vi "Recipe.vi"() -> ()   [LabVIEW 2020, in "SMCD14_lib.lvlib"]
uses:
  SMCD14_lib.lvlib
  Macro Cluster.ctl
  typedefAxisConfiguration.ctl
  ConnectionData.vi
  AxisWriteValues.vi
  AxisWriteValues_Write.vi
panel:
  out "AxisBaseAddr":u16[](array[numeric])
  in  "Macro Table":T1[](array[typedef]) {"M5_select_action" items=["Stop", "Safe Position", "Working Position", "Run scaning", "Transfer posituin"]; "SelectedTargetCtrl" items=["none", "Target 1", "Target 2", "Target 3", "Target 4", "Target 5", "Target 6", "Laser test"]; "M3_Type" items=["Type1", "Type2", "Type3", "Type4", "Type5"]; "M3_1_Time" format="%<%H:%M:%S>t"; "MoveModeControl" items=["Absolute"=1, "Relative"=2, "Velocity"=3, "Homing"=4, "none"=0]; "M2_Target_Vel" format="%<%H:%M:%S>t"; "M2_Axis" items=["Axis no1", "Axis no2", "Axis no3", "Axis no4", "Axis no5", "Axis no6"]; "M1_action_axis 6" items=["NONE", "Start", "Stop", "Clear", "Motor ON", "motor OFF"]; "M1_action_axis 5" items=["NONE", "Start", "Stop", "Clear", "Motor ON", "motor OFF"]; "M1_action_axis 4" items=["NONE", "Start", "Stop", "Clear", "Motor ON", "motor OFF"]; "M1_action_axis 3" items=["------", "Manual", "Time SP", "Thickness SP"]; "M1_action_axis 2" items=["NONE", "Start", "Stop", "Clear", "Motor ON", "motor OFF"]; "M1_action_axis 1" items=["NONE", "Start", "Stop", "Clear", "Motor ON", "motor OFF"]; "Macro Type" items=["Action", "Parameters", "Wait"]}
  out "AxisNames":string[](array[string])
  out "Recipe example":refnum<vi>
  in  "AxisControlSubPanelRefArray":refnum<vi>[](array[refnum])
  in  "AxesCount":i32=6
  out "AllowCalib":bool
  out "Act. macro:":string
  out "Recipe Finish:":bool
  out "Recipe in Progress:":bool
  out "?":cluster{dbl, dbl}(slide)={-100.0, 0.0} scale=0.0..100.0 scale format="%.0f %"
  out "Act. Step:":i32=-1
  in  "Stop Recipe":bool
  in  "Start Recipe":bool
  in  "Next macro":bool
  in  "E. Recipe":bool=TRUE
  out "MacroStart Time":timestamp
  out "Act. Macro:":i32=-1
  out "SlavesID":u16[](array[numeric])
  out "size":i32=1
  out "New Macro":bool
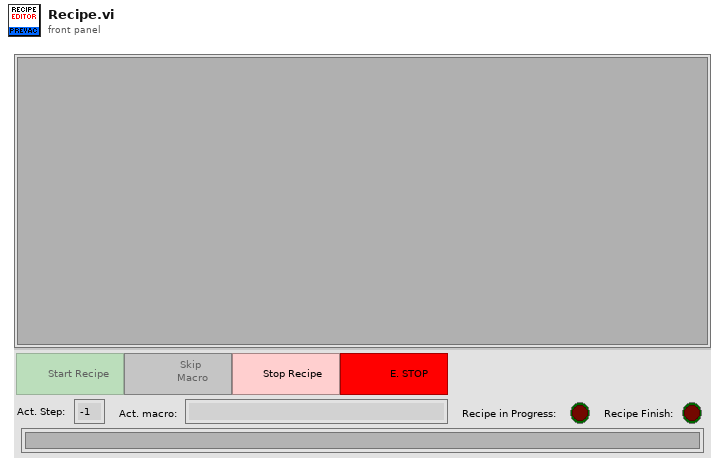
[diagram p1: front panel]
types:
  T1 = typedef "SMCD14_lib.lvlib/Macro Cluster.ctl" = cluster{"Macro Type":u16, "Macro Name":string, "Macro Description":string, "M1_action_axis 1":u16, "M1_action_axis 2":u16, "M1_action_axis 3":u16, "M1_action_axis 4":u16, "M1_action_axis 5":u16, "M1_action_axis 6":u16, "M2_Axis":u16, "M2_Target_Pos":sgl, "M2_Target_Vel":sgl, "MoveModeControl":u16, "M3_1_Time":u32, "M3_Type":u16, "M3_2_wait_for_axis 1":bool, "M3_2_wait_for_axis 2":bool, "M3_2_wait_for_axis 3":bool, "M3_2_wait_for_axis 4":bool, "M3_2_wait_for_axis 5":bool, "M3_2_wait_for_axis 6":bool, "M3_3_mesage":string, "M3_3_wait_for_calib":bool, "SelectedTargetCtrl":u16, "M5_select_action":u16}
  T2 = typedef "SMCD14_lib.lvlib/AxisWriteValues_typedef.ctl" = cluster{"AxisTarget":dbl, "AxisTargetVel":dbl, "AxisStartReq":bool, "AxisStopReq":bool, "AxisClearReq":bool, "AxisMovetype":bool, "AxisMotorON":bool, "MoveModeControl":u16, "AxisHomingVel":dbl, "AxisAccDecc":dbl}
  T3 = enum16{"Left Button", "Center Button", "Right Button", "Window Close"}
  T4 = enum8{"Enabled", "Disabled", "Disabled and Grayed Out"}
  T5 = typedef "SMCD14_lib.lvlib/ConnectionData_typedef.ctl" = cluster{"DeviceIDCtrl":u16, "ProtocolCtrl":enum16{"Modbus RTU", "Modbus TCP", ""}, "COMportCtrl":refnum<visa-resource-name>, "IPCtrl":string, "serial master instance":refnum<class "Modbus Master.lvclass">, "ConnectionStatusIndicator":bool}
  T6 = typedef "SMCD14_lib.lvlib/typedefAxisConfiguration.ctl" = cluster{"AxisName":string, "UnitsControl":u16, "AxisSlaveID":u16, "AxisBaseAddr":u16, "AxisMinSpeed":dbl, "AxisMaxSpeed":dbl}
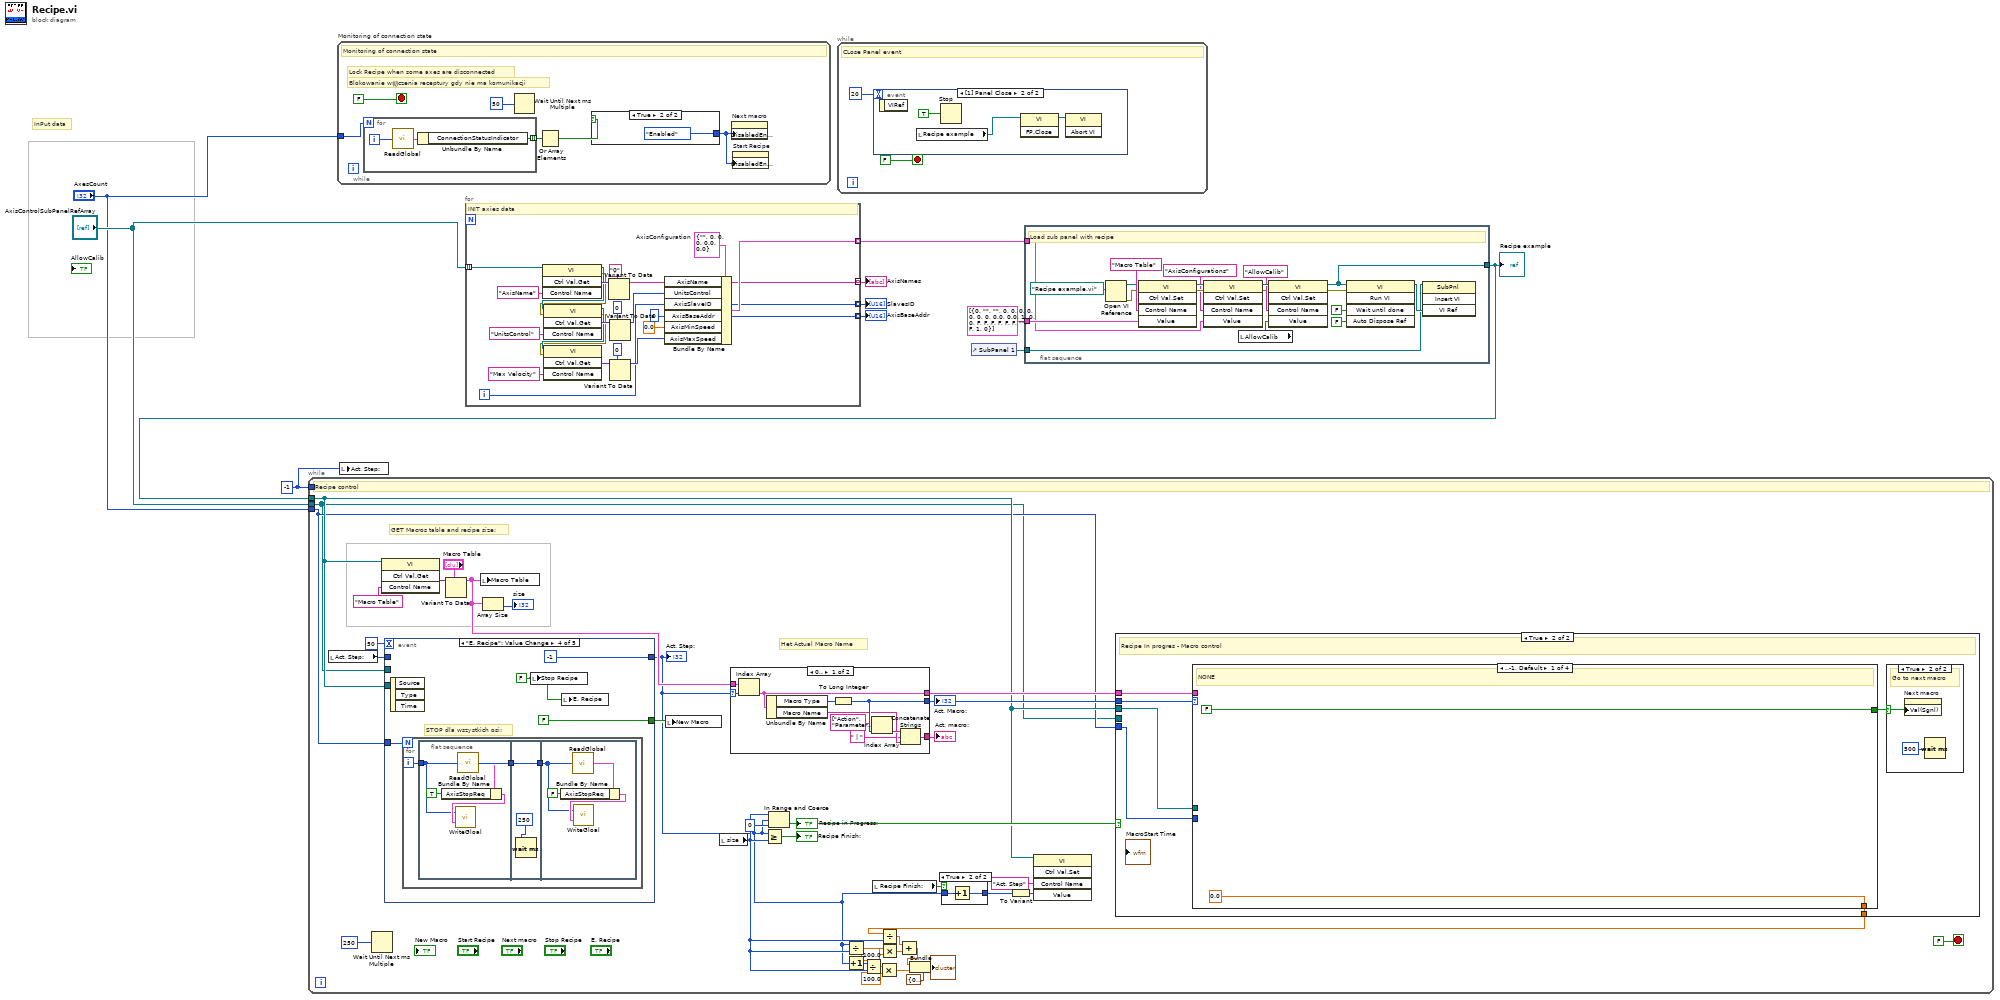
[diagram p0: block diagram]
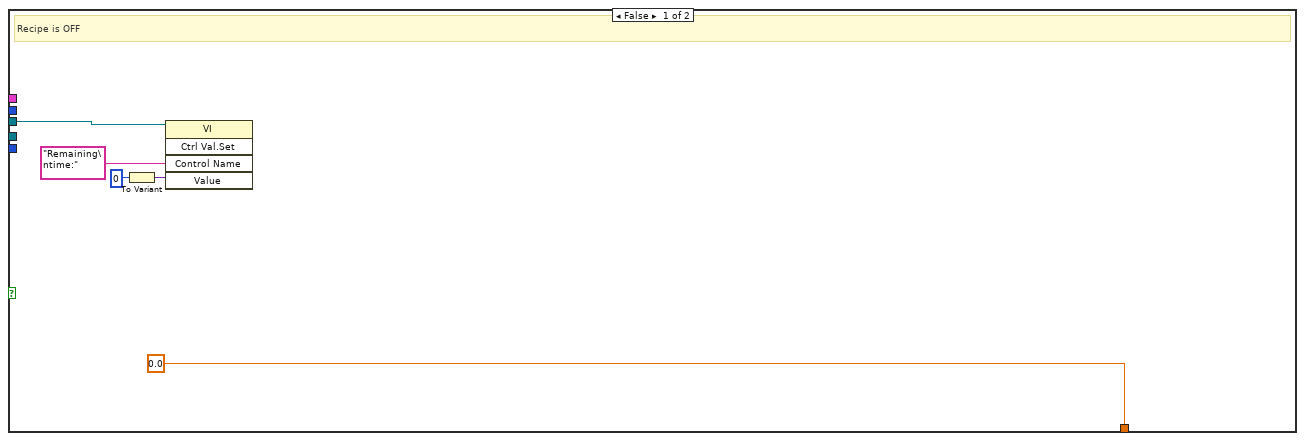
[diagram p3: hidden frame]
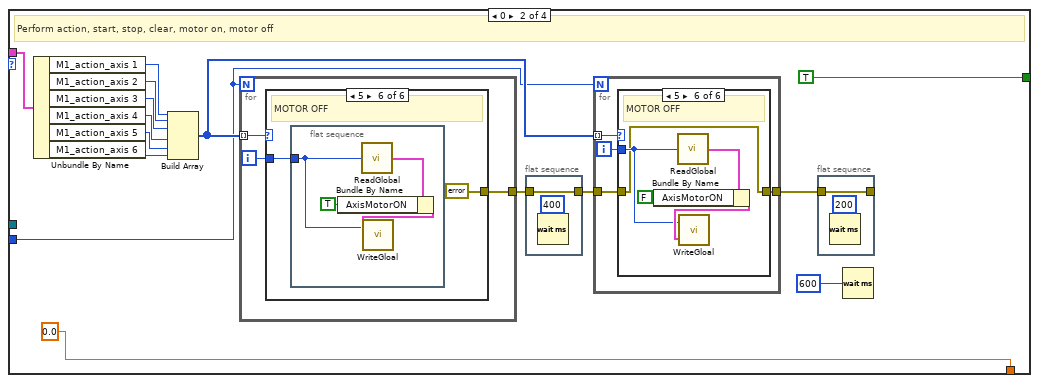
[diagram p5: hidden frame]
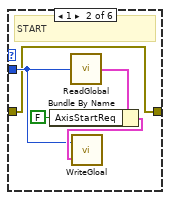
[diagram p7: hidden frame]
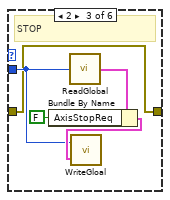
[diagram p8: hidden frame]
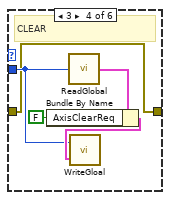
[diagram p9: hidden frame]
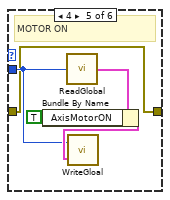
[diagram p10: hidden frame]
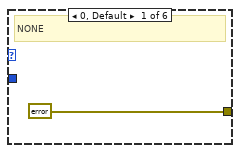
[diagram p11: hidden frame]
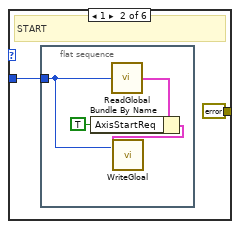
[diagram p12: hidden frame]
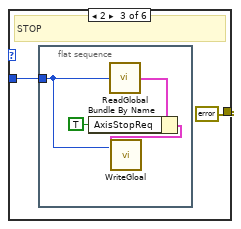
[diagram p13: hidden frame]
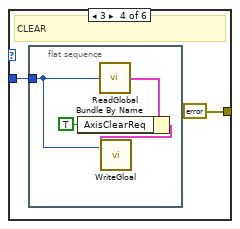
[diagram p14: hidden frame]
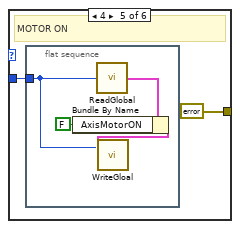
[diagram p15: hidden frame]
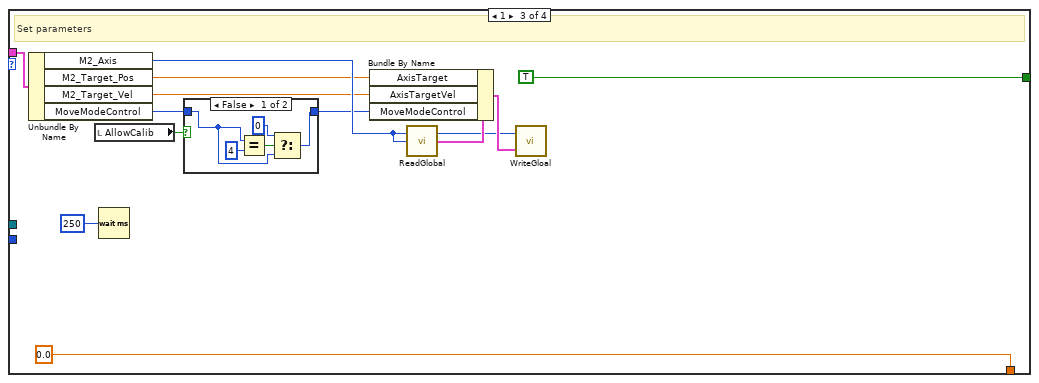
[diagram p16: hidden frame]
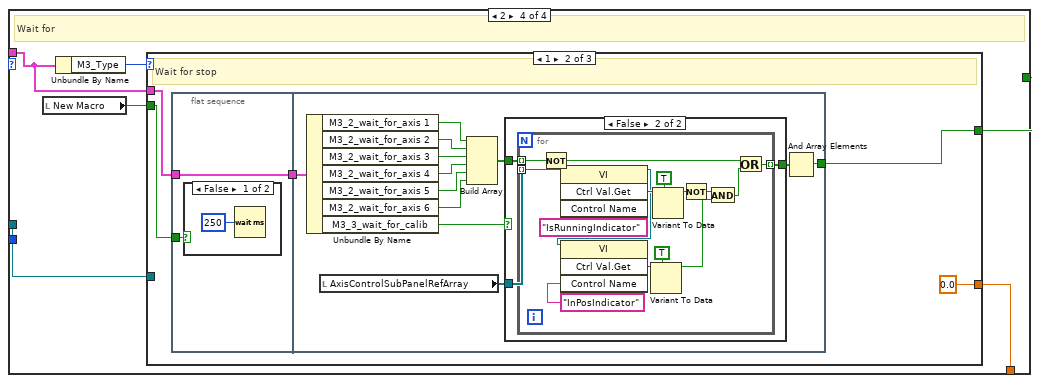
[diagram p18: hidden frame]
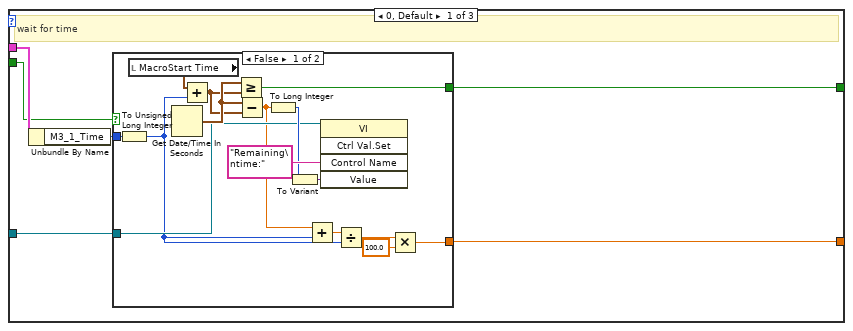
[diagram p19: hidden frame]
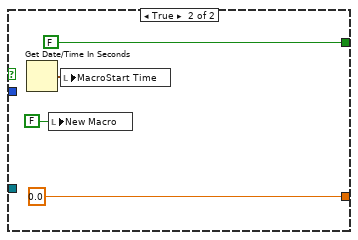
[diagram p20: hidden frame]
diagram:
  w7 = -1
  # "InPut data"
  n1 = while {
    tunnel: w4 -> [w15]
    tunnel: w7 -> [_]
    tunnel: "AxisControlSubPanelRefArray" -> [w11]
    tunnel: "AxesCount" -> [w12]
    stop <- FALSE stop-if-true
    # "Het Actual Macro Name"
    # "GET Macros table and recipe size:"
    # "Recipe control"
    n2 = local read "Act. Step:"() -> (w46:i32)
    n3 = Wait Until Next ms Multiple(millisecond multiple=u32 250) -> ()  [unwired: 1 out]
    n4 = invoke class="VI" method="Ctrl Val.Get"(reference=w15, "Control Name"="Macro Table") -> ("Get Control Value Variant"=w40:variant)  [unwired: 2 in, 3 out]
    n5 = event shown="[3] \"E. Recipe\": Value Change" {
      selector: _ -> [_ _ _ _ _]
      dyn-events: _ -> [_ _ _ _ _]
      timeout: 50 -> [_ _ _ _ _]
      tunnel: w46 -> [w281 _ _ _ w314]
      tunnel: [w280 0 ("millisecond multiple") -1 ("millisecond multiple") -1 ("millisecond multiple") w312] -> w13
      tunnel: [w287 TRUE ("Play Button") FALSE ("Play Button") FALSE ("Play Button") TRUE ("New Macro")] -> w43
      tunnel: w11 -> [_ _ _ _ _]
      tunnel: w15 -> [w284 _ _ _ _]
      tunnel: w12 -> [_ _ _ w294 _]
      event Timeout {
        n6 = event-data() -> ()  [unwired: 1 in, 3 out]
        n7 = local read "Recipe in Progress:"() -> (w279:bool)
        n8 = invoke class="VI" method="Ctrl Val.Get"(reference=w284, "Control Name"="edit?") -> ("Get Control Value Variant"=w286:variant)  [unwired: 2 in, 3 out]
        n9 = Variant To Data(type=FALSE ("Play Button"), Variant=w286) -> (data=w277:bool)  [unwired: 1 in, 1 out]
        n10 = Not(x=w279) -> (.not. x?=w278:bool)
        n11 = local read "New Macro"() -> (w287:bool)
        n12 = And(x=w278, y=w277) -> (x .and. y?=w276:bool)
        n13 = Select(t=-1, s=w276, f=w281) -> (s? t:f=w280:i32)
      }
      event "Start Recipe": Value Change {
        n14 = event-data() -> ()  [unwired: 1 in, 3 out]
        n15 = local write "Start Recipe"(FALSE ("Play Button")) -> ()
      }
      event "Stop Recipe": Value Change {
        n16 = event-data() -> ()  [unwired: 1 in, 3 out]
        n17 = local write "Stop Recipe"(FALSE ("Play Button")) -> ()
      }
      event "E. Recipe": Value Change {
        w295 = FALSE ("Play Button")
        # "STOP dla wszystkich osi:"
        n18 = event-data() -> ()  [unwired: 1 in, 3 out]
        n19 = for {
          N: w294 -> [_]
          i -> [w298]
          n20 = flat-sequence {
            tunnel: w298 -> [w302]
            tunnel: [w302] -> w300
            tunnel: w300 -> [w305]
            tunnel: [w305] -> w299
            tunnel: w299 -> [w307]
            frame #0 {
              n21 = call-poly "ReadGlobal.vi"("AxisNo"=w302) -> ("AxisWriteValuesOUT"=w301:T2)
              n22 = Bundle By Name(cluster=w301, "AxisStopReq"=TRUE ("AxisWriteValues.AxisMotorON")) -> (w303:T2)
              n23 = call-poly "WriteGloal.vi"("AxisWriteValuesIN"=w303, "AxisNo"=w302) -> ()  [unwired: 1 in]
            }
            frame #1 {
              n24 = Wait (ms)(milliseconds to wait=u32 250) -> ()  [unwired: 1 out]
            }
            frame #2 {
              n25 = call-poly "ReadGlobal.vi"("AxisNo"=w307) -> ("AxisWriteValuesOUT"=w309:T2)
              n26 = Bundle By Name(cluster=w309, "AxisStopReq"=FALSE ("AxisWriteValues.AxisMotorON")) -> (w308:T2)
              n27 = call-poly "WriteGloal.vi"("AxisWriteValuesIN"=w308, "AxisNo"=w307) -> ()  [unwired: 1 in]
            }
          }
        }
        n28 = local write "Stop Recipe"(w295) -> ()
        n29 = local write "E. Recipe"(w295) -> ()
      }
      event "Next macro": Value Change {
        n30 = event-data() -> ()  [unwired: 1 in, 1 out]
        n31 = Greater Or Equal To 0?(x=w314) -> (x >= 0?=w318:bool)
        n32 = local read "size"() -> (w313:i32)
        n33 = case shown="True" w318 {
          tunnel: [w320 w322] -> w316
          tunnel: w314 -> [w320 w321]
          frame False {
          }
          frame True {
            n34 = Increment(x=w321) -> (x+1=w322:i32)
          }
        }
        n35 = Increment(x=w313) -> (x+1=w317:i32)
        n36 = In Range and Coerce(upper limit=w317, x=w316, lower limit=0 ("millisecond multiple")) -> (coerced(x)=w312:i32)  [unwired: 1 out]
        n37 = local write "Next macro"(FALSE ("Play Button")) -> ()
      }
    }
    "Act. Step:" <- w13
    n38 = Variant To Data(type="Macro Table", Variant=w40) -> (data=w26:T1[])  [unwired: 1 in, 1 out]
    n39 = local write "Macro Table"(w26) -> ()
    n40 = Array Size(array=w26) -> (size(s)=→"size":i32)
    n41 = local write "New Macro"(w43) -> ()
    n42 = local read "size"() -> (w14:i32)
    n43 = case shown="0.." w13 {
      selector: w13 -> [w272 _]
      tunnel: [w269 T1 {"Macro Type"=0, "Macro Name"="", "Macro Description"="", "M1_action_axis 1"=0, "M1_action_axis 2"=0, "M1_action_axis 3"=0, "M1_action_axis 4"=0, "M1_action_axis 5"=0, "M1_action_axis 6"=0, "M2_Axis"=0, "M2_Target_Pos"=0.0, "M2_Target_Vel"=0.0, "MoveModeControl"=0, "M3_1_Time"=0, "M3_Type"=0, "M3_2_wait_for_axis 1"=FALSE, "M3_2_wait_for_axis 2"=FALSE, "M3_2_wait_for_axis 3"=FALSE, "M3_2_wait_for_axis 4"=FALSE, "M3_2_wait_for_axis 5"=FALSE, "M3_2_wait_for_axis 6"=FALSE, "M3_3_mesage"="", "M3_3_wait_for_calib"=FALSE, "SelectedTargetCtrl"=1, "M5_select_action"=0} ("Macro Cluster")] -> w28
      tunnel: [w268 -1 ("millisecond multiple")] -> w25
      tunnel: w26 -> [w271 _]
      tunnel: [w263 "" ("Macro Name")] -> w24
      frame 0.. {
        n44 = Index Array(array=w271, index=w272) -> (element=w269:T1)
        n45 = Unbundle By Name(w269) -> ("Macro Type"=w270:u16, "Macro Name"=w265:string)
        n46 = To Long Integer(number=w270) -> (32bit integer=w268:i32)
        n47 = Index Array(array=string[] ["Action", "Parameters", "Wait"], index=w268) -> (element=w266:string)
        n48 = Concatenate Strings(w266, " | " ("string"), w265) -> (w263:string)
      }
      frame ..-1, Default {
      }
    }
    "Act. Macro:" <- w25
    "Act. macro:" <- w24
    n49 = Greater Or Equal?(x=w13, y=w14) -> (x >= y?=→"Recipe Finish:":bool)
    n50 = In Range and Coerce(upper limit=w14, x=w13, lower limit=0 ("millisecond multiple")) -> (In Range?=w29:bool)  [unwired: 1 out]
    "Recipe in Progress:" <- w29
    n51 = Divide(x=w13, y=w14) -> (x/y=w39:dbl)
    n52 = Increment(x=w13) -> (x+1=w33:i32)
    n53 = Divide(x=w33, y=w14) -> (x/y=w34:dbl)
    n54 = local read "Recipe Finish:"() -> (w17:bool)
    n55 = Multiply(x=w34, y=100.0) -> (x*y=w31:dbl)
    n56 = Multiply(x=w39, y=100.0) -> (x*y=w23:dbl)
    n57 = case shown="True" w17 {
      tunnel: w13 -> [w48 w50]
      tunnel: [w48 w49] -> w16
      frame False {
      }
      frame True {
        n58 = Increment(x=w50) -> (x+1=w49:i32)
      }
    }
    n59 = To Variant(anything=w16) -> (Variant=w19:variant)
    n60 = invoke class="VI" method="Ctrl Val.Set"(reference=w15, "Control Name"="Act. Step", "Value"=w19) -> ()  [unwired: 2 in, 5 out]
    n61 = case shown="True" w29 {
      tunnel: w28 -> [_ w59]
      tunnel: w25 -> [_ w61]
      tunnel: w15 -> [w52 w58]
      tunnel: [0.0 ("y") w57] -> w21
      tunnel: w12 -> [_ w56]
      tunnel: w11 -> [_ _]
      frame False {
        # "Recipe is OFF"
        n62 = To Variant(anything=0) -> (Variant=w55:variant)
        n63 = invoke class="VI" method="Ctrl Val.Set"(reference=w52, "Control Name"="Remaining\ntime:", "Value"=w55) -> ()  [unwired: 2 in, 5 out]
      }
      frame True {
        # "Recipe In progres - Macro control"
        n64 = case shown="..-1, Default" w61 {
          tunnel: [FALSE ("true") TRUE TRUE w167] -> w60
          tunnel: w59 -> [_ w80 w160 w170]
          tunnel: w58 -> [_ _ _ w169]
          tunnel: [0.0 0.0 0.0 w168] -> w57
          tunnel: w56 -> [_ w69 _ _]
          frame ..-1, Default {
            # "NONE"
          }
          frame 0 {
            # "Perform action, start, stop, clear, motor on, motor off"
            n65 = Unbundle By Name(w80) -> ("M1_action_axis 1"=w79:u16, "M1_action_axis 2"=w78:u16, "M1_action_axis 3"=w77:u16, "M1_action_axis 4"=w76:u16, "M1_action_axis 5"=w75:u16, "M1_action_axis 6"=w74:u16)
            n66 = Build Array(w79, w78, w77, w76, w75, w74) -> (w71:u16[])
            n67 = for {
              N: w69 -> [_]
              tunnel: w71 -> [w117] mode=indexing
              tunnel: [w116] -> w68
              i -> [w115]
              n68 = case shown="5" w117 {
                tunnel: [errorcluster {"status"=FALSE, "code"=0, "source"=""} ("error out") errorcluster {"status"=FALSE, "code"=0, "source"=""} ("error out") errorcluster {"status"=FALSE, "code"=0, "source"=""} ("error out") errorcluster {"status"=FALSE, "code"=0, "source"=""} ("error out") errorcluster {"status"=FALSE, "code"=0, "source"=""} ("error out") errorcluster {"status"=FALSE, "code"=0, "source"=""} ("error out")] -> w116
                tunnel: w115 -> [_ w120 w126 w132 w138 w144]
                frame 0, Default {
                  # "NONE"
                }
                frame 1 {
                  # "START"
                  n69 = flat-sequence {
                    tunnel: w120 -> [w121]
                    frame #0 {
                      n70 = call-poly "ReadGlobal.vi"("AxisNo"=w121) -> ("AxisWriteValuesOUT"=w123:T2)
                      n71 = Bundle By Name(cluster=w123, "AxisStartReq"=TRUE ("AxisWriteValues.AxisMotorON")) -> (w122:T2)
                      n72 = call-poly "WriteGloal.vi"("AxisWriteValuesIN"=w122, "AxisNo"=w121) -> ()  [unwired: 1 in]
                    }
                  }
                }
                frame 2 {
                  # "STOP"
                  n73 = flat-sequence {
                    tunnel: w126 -> [w127]
                    frame #0 {
                      n74 = call-poly "ReadGlobal.vi"("AxisNo"=w127) -> ("AxisWriteValuesOUT"=w129:T2)
                      n75 = Bundle By Name(cluster=w129, "AxisStopReq"=TRUE ("AxisWriteValues.AxisMotorON")) -> (w128:T2)
                      n76 = call-poly "WriteGloal.vi"("AxisWriteValuesIN"=w128, "AxisNo"=w127) -> ()  [unwired: 1 in]
                    }
                  }
                }
                frame 3 {
                  # "CLEAR"
                  n77 = flat-sequence {
                    tunnel: w132 -> [w133]
                    frame #0 {
                      n78 = call-poly "ReadGlobal.vi"("AxisNo"=w133) -> ("AxisWriteValuesOUT"=w135:T2)
                      n79 = Bundle By Name(cluster=w135, "AxisClearReq"=TRUE ("AxisWriteValues.AxisMotorON")) -> (w134:T2)
                      n80 = call-poly "WriteGloal.vi"("AxisWriteValuesIN"=w134, "AxisNo"=w133) -> ()  [unwired: 1 in]
                    }
                  }
                }
                frame 4 {
                  # "MOTOR ON"
                  n81 = flat-sequence {
                    tunnel: w138 -> [w139]
                    frame #0 {
                      n82 = call-poly "ReadGlobal.vi"("AxisNo"=w139) -> ("AxisWriteValuesOUT"=w141:T2)
                      n83 = Bundle By Name(cluster=w141, "AxisMotorON"=FALSE ("AxisWriteValues.AxisMotorON")) -> (w140:T2)
                      n84 = call-poly "WriteGloal.vi"("AxisWriteValuesIN"=w140, "AxisNo"=w139) -> ()  [unwired: 1 in]
                    }
                  }
                }
                frame 5 {
                  # "MOTOR OFF"
                  n85 = flat-sequence {
                    tunnel: w144 -> [w145]
                    frame #0 {
                      n86 = call-poly "ReadGlobal.vi"("AxisNo"=w145) -> ("AxisWriteValuesOUT"=w147:T2)
                      n87 = Bundle By Name(cluster=w147, "AxisMotorON"=TRUE ("AxisWriteValues.AxisMotorON")) -> (w146:T2)
                      n88 = call-poly "WriteGloal.vi"("AxisWriteValuesIN"=w146, "AxisNo"=w145) -> ()  [unwired: 1 in]
                    }
                  }
                }
              }
            }
            n89 = flat-sequence {
              tunnel: w68 -> [w83]
              tunnel: [w83] -> w67
              frame #0 {
                n90 = Wait (ms)(milliseconds to wait=u32 400) -> ()  [unwired: 1 out]
              }
            }
            n91 = for {
              N: w69 -> [_]
              tunnel: w71 -> [w88] mode=indexing
              tunnel: w67 -> [w87]
              tunnel: [w86] -> w66
              i -> [w85]
              n92 = case shown="5" w88 {
                tunnel: w87 -> [w89 w90 w95 w100 w105 w110]
                tunnel: [w89 w90 w95 w100 w105 w110] -> w86
                tunnel: w85 -> [_ w91 w96 w101 w106 w111]
                frame 0, Default {
                  # "NONE"
                }
                frame 1 {
                  # "START"
                  n93 = call-poly "ReadGlobal.vi"("AxisNo"=w91) -> ("AxisWriteValuesOUT"=w93:T2)
                  n94 = Bundle By Name(cluster=w93, "AxisStartReq"=FALSE ("AxisWriteValues.AxisMotorON")) -> (w92:T2)
                  n95 = call-poly "WriteGloal.vi"("AxisWriteValuesIN"=w92, "AxisNo"=w91) -> ()  [unwired: 1 in]
                }
                frame 2 {
                  # "STOP"
                  n96 = call-poly "ReadGlobal.vi"("AxisNo"=w96) -> ("AxisWriteValuesOUT"=w98:T2)
                  n97 = Bundle By Name(cluster=w98, "AxisStopReq"=FALSE ("AxisWriteValues.AxisMotorON")) -> (w97:T2)
                  n98 = call-poly "WriteGloal.vi"("AxisWriteValuesIN"=w97, "AxisNo"=w96) -> ()  [unwired: 1 in]
                }
                frame 3 {
                  # "CLEAR"
                  n99 = call-poly "ReadGlobal.vi"("AxisNo"=w101) -> ("AxisWriteValuesOUT"=w103:T2)
                  n100 = Bundle By Name(cluster=w103, "AxisClearReq"=FALSE ("AxisWriteValues.AxisMotorON")) -> (w102:T2)
                  n101 = call-poly "WriteGloal.vi"("AxisWriteValuesIN"=w102, "AxisNo"=w101) -> ()  [unwired: 1 in]
                }
                frame 4 {
                  # "MOTOR ON"
                  n102 = call-poly "ReadGlobal.vi"("AxisNo"=w106) -> ("AxisWriteValuesOUT"=w108:T2)
                  n103 = Bundle By Name(cluster=w108, "AxisMotorON"=TRUE ("AxisWriteValues.AxisMotorON")) -> (w107:T2)
                  n104 = call-poly "WriteGloal.vi"("AxisWriteValuesIN"=w107, "AxisNo"=w106) -> ()  [unwired: 1 in]
                }
                frame 5 {
                  # "MOTOR OFF"
                  n105 = call-poly "ReadGlobal.vi"("AxisNo"=w111) -> ("AxisWriteValuesOUT"=w113:T2)
                  n106 = Bundle By Name(cluster=w113, "AxisMotorON"=FALSE ("AxisWriteValues.AxisMotorON")) -> (w112:T2)
                  n107 = call-poly "WriteGloal.vi"("AxisWriteValuesIN"=w112, "AxisNo"=w111) -> ()  [unwired: 1 in]
                }
              }
            }
            n108 = flat-sequence {
              tunnel: w66 -> [w81]
              tunnel: [w81] -> _
              frame #0 {
                n109 = Wait (ms)(milliseconds to wait=u32 200) -> ()  [unwired: 1 out]
              }
            }
            n110 = Wait (ms)(milliseconds to wait=u32 600) -> ()  [unwired: 1 out]
          }
          frame 1 {
            # "Set parameters"
            n111 = Unbundle By Name(w160) -> ("M2_Axis"=w152:u16, "M2_Target_Pos"=w151:sgl, "M2_Target_Vel"=w150:sgl, "MoveModeControl"=w155:u16)
            n112 = local read "AllowCalib"() -> (w156:bool)
            n113 = Wait (ms)(milliseconds to wait=u32 250) -> ()  [unwired: 1 out]
            n114 = case shown="False" w156 {
              tunnel: w155 -> [w162 w166]
              tunnel: [w161 w166] -> w149
              frame False {
                n115 = Equal?(x=w162, y=u16 4 ("MoveModeControl")) -> (x = y?=w164:bool)
                n116 = Select(t=u16 0 ("MoveModeControl"), s=w164, f=w162) -> (s? t:f=w161:u16)
              }
              frame True {
              }
            }
            n117 = call-poly "ReadGlobal.vi"("AxisNo"=w152) -> ("AxisWriteValuesOUT"=w154:T2)
            n118 = Bundle By Name(cluster=w154, "AxisTarget"=w151, "AxisTargetVel"=w150, "MoveModeControl"=w149) -> (w153:T2)
            n119 = call-poly "WriteGloal.vi"("AxisWriteValuesIN"=w153, "AxisNo"=w152) -> ()  [unwired: 1 in]
          }
          frame 2 {
            # "Wait for"
            n120 = local read "New Macro"() -> (w171:bool)
            n121 = Unbundle By Name(w170) -> ("M3_Type"=w172:u16)
            n122 = case shown="1" w172 {
              tunnel: [w175 w201 w249] -> w167
              tunnel: w171 -> [w177 w198 _]
              tunnel: w170 -> [w178 w202 w256]
              tunnel: w169 -> [w174 _ _]
              tunnel: [w173 0.0 0.0] -> w168
              frame 0, Default {
                # "wait for time"
                n123 = Unbundle By Name(w178) -> ("M3_1_Time"=w176:u32)
                n124 = case shown="False" w177 {
                  tunnel: w176 -> [w192 _]
                  tunnel: [w191 FALSE ("New Macro")] -> w175
                  tunnel: w174 -> [w185 _]
                  tunnel: [w179 0.0] -> w173
                  frame False {
                    n125 = To Unsigned Long Integer(number=w192) -> (unsigned 32bit integer=w182:u32)
                    n126 = local read "MacroStart Time"() -> (w193:timestamp)
                    n127 = Get Date/Time In Seconds() -> (seconds since 1Jan1904=w190:timestamp)
                    n128 = Add(x=w193, y=w182) -> (x+y=w189:timestamp)
                    n129 = Greater Or Equal?(x=w190, y=w189) -> (x >= y?=w191:bool)
                    n130 = Subtract(x=w190, y=w189) -> (x-y=w184:dbl)
                    n131 = To Long Integer(number=w184) -> (32bit integer=w186:i32)
                    n132 = To Variant(anything=w186) -> (Variant=w188:variant)
                    n133 = Add(x=w184, y=w182) -> (x+y=w183:dbl)
                    n134 = invoke class="VI" method="Ctrl Val.Set"(reference=w185, "Control Name"="Remaining\ntime:", "Value"=w188) -> ()  [unwired: 2 in, 5 out]
                    n135 = Divide(x=w183, y=w182) -> (x/y=w180:dbl)
                    n136 = Multiply(x=w180, y=100.0) -> (x*y=w179:dbl)
                  }
                  frame True {
                    n137 = Get Date/Time In Seconds() -> (seconds since 1Jan1904=w197:timestamp)
                    n138 = local write "New Macro"(FALSE ("New Macro")) -> ()
                    n139 = local write "MacroStart Time"(w197) -> ()
                  }
                }
              }
              frame 1 {
                # "Wait for stop"
                n140 = flat-sequence {
                  tunnel: w202 -> [w204]
                  tunnel: [w204] -> w199
                  tunnel: w198 -> [w203]
                  tunnel: [w208] -> w201
                  tunnel: w199 -> [w218]
                  frame #0 {
                    n141 = case shown="False" w203 {
                      frame False {
                        n142 = Wait (ms)(milliseconds to wait=u32 250) -> ()  [unwired: 1 out]
                      }
                      frame True {
                        n143 = Wait (ms)(milliseconds to wait=u32 1500) -> ()  [unwired: 1 out]
                      }
                    }
                  }
                  frame #1 {
                    n144 = Unbundle By Name(w218) -> ("M3_2_wait_for_axis 1"=w217:bool, "M3_2_wait_for_axis 2"=w216:bool, "M3_2_wait_for_axis 3"=w215:bool, "M3_2_wait_for_axis 4"=w214:bool, "M3_2_wait_for_axis 5"=w213:bool, "M3_2_wait_for_axis 6"=w212:bool, "M3_3_wait_for_calib"=w207:bool)
                    n145 = local read "AxisControlSubPanelRefArray"() -> (w210:refnum<vi>[])
                    n146 = Build Array(w217, w216, w215, w214, w213, w212) -> (w211:bool[])
                    n147 = case shown="False" w207 {
                      tunnel: w211 -> [w220 w232]
                      tunnel: w210 -> [w221 w231]
                      tunnel: [w219 w230] -> w209
                      frame True {
                        n148 = for {
                          tunnel: w221 -> [w226] mode=indexing
                          tunnel: w220 -> [w225] mode=indexing
                          tunnel: [w222] -> w219 mode=indexing
                          n149 = invoke class="VI" method="Ctrl Val.Get"(reference=w226, "Control Name"="IsHomedIndicator") -> ("Get Control Value Variant"=w227:variant)  [unwired: 2 in, 3 out]
                          n150 = Not(x=w225) -> (.not. x?=w224:bool)
                          n151 = Variant To Data(type=TRUE, Variant=w227) -> (data=w223:bool)  [unwired: 1 in, 1 out]
                          n152 = Or(x=w224, y=w223) -> (x .or. y?=w222:bool)
                        }
                      }
                      frame False {
                        n153 = for {
                          tunnel: w232 -> [w238] mode=indexing
                          tunnel: [w233] -> w230 mode=indexing
                          tunnel: w231 -> [w247] mode=indexing
                          n154 = Not(x=w238) -> (.not. x?=w235:bool)
                          n155 = invoke class="VI" method="Ctrl Val.Get"(reference=w247, "Control Name"="IsRunningIndicator") -> (reference out=w243:refnum<vi>, "Get Control Value Variant"=w244:variant)  [unwired: 2 in, 2 out]
                          n156 = invoke class="VI" method="Ctrl Val.Get"(reference=w243, "Control Name"="InPosIndicator") -> ("Get Control Value Variant"=w241:variant)  [unwired: 2 in, 3 out]
                          n157 = Variant To Data(type=TRUE, Variant=w241) -> (data=w239:bool)  [unwired: 1 in, 1 out]
                          n158 = Variant To Data(type=TRUE, Variant=w244) -> (data=w237:bool)  [unwired: 1 in, 1 out]
                          n159 = Not(x=w237) -> (.not. x?=w236:bool)
                          n160 = And(x=w236, y=w239) -> (x .and. y?=w234:bool)
                          n161 = Or(x=w235, y=w234) -> (x .or. y?=w233:bool)
                        }
                      }
                    }
                    n162 = And Array Elements(Boolean array=w209) -> (logical AND=w208:bool)
                  }
                }
              }
              frame 2 {
                # "Wait for action"
                n163 = Unbundle By Name(w256) -> ("M3_3_mesage"=w251:string)
                n164 = call <vilib>:"Three Button Dialog.vi"("Window Title (\"\")"="Wait for user action" ("message"), "Right Button Text (\"Cancel\")"="E. STOP" ("F button name (\"Cancel\")"), "Center Button Text (\"No\")"="Stop recipe" ("F button name (\"Cancel\")"), "Left Button Text (\"Yes\")"="OK - Go to next step" ("T button name (\"OK\")"), "message"=w251) -> ("Which Button?"=w250:T3)  [unwired: 6 in]
                n165 = case shown="\"Center Button\"" w250 {
                  tunnel: [TRUE FALSE FALSE FALSE] -> w249
                  frame "Left Button", Default {
                  }
                  frame "Center Button" {
                    n166 = property on="Stop Recipe" class="Bool (strict)"("Val(Sgnl)"=TRUE) -> ()  [unwired: 2 in, 2 out]
                  }
                  frame "Right Button" {
                    n167 = property on="E. Recipe" class="Bool (strict)"("Val(Sgnl)"=FALSE) -> ()  [unwired: 2 in, 2 out]
                  }
                  frame "Window Close" {
                  }
                }
              }
            }
          }
        }
        n168 = case shown="True" w60 {
          selector: w60 -> [_ w63]
          frame False {
          }
          frame True {
            # "Go to next macro"
            n169 = property on="Next macro" class="Bool (strict)"("Val(Sgnl)"=w63) -> ()  [unwired: 2 in, 2 out]
            n170 = Wait (ms)(milliseconds to wait=u32 500) -> ()  [unwired: 1 out]
          }
        }
      }
    }
    n171 = Divide(x=w21, y=w14) -> (x/y=w20:dbl)
    n172 = Add(x=w20, y=w23) -> (x+y=w22:dbl)
    n173 = Bundle(cluster=cluster{dbl, dbl} {0.0, 0.0}, w22, w31) -> (→"?":cluster{dbl, dbl})
  }
  n174 = while "Monitoring of connection state" {
    tunnel: "AxesCount" -> [w323]
    stop <- FALSE stop-if-true
    # "Lock Recipe when some axes are disconnected"
    # "Blokowanie w彻czenia receptury gdy nie ma komunikacji"
    # "Monitoring of connection state"
    n175 = for {
      N: w323 -> [_]
      tunnel: [w330] -> w325 mode=indexing
      i -> [w329]
      n176 = call-poly "ReadGlobal.vi"("AxisNo"=w329) -> ("ConnectionDataOUT"=w331:T5)
      n177 = Unbundle By Name(w331) -> ("ConnectionStatusIndicator"=w330:bool)
    }
    n178 = Wait Until Next ms Multiple(millisecond multiple=u32 50) -> ()  [unwired: 1 out]
    n179 = Or Array Elements(Boolean array=w325) -> (logical OR=w324:bool)
    n180 = case shown="True" w324 {
      tunnel: [T4."Disabled and Grayed Out" ("Disabled") T4."Enabled" ("Disabled")] -> w326
      frame False {
      }
      frame True {
      }
    }
    n181 = property on="Next macro" class="Bool (strict)"("DisabledEnum"=w326) -> ()  [unwired: 2 in, 2 out]
    n182 = property on="Start Recipe" class="Bool (strict)"("DisabledEnum"=w326) -> ()  [unwired: 2 in, 2 out]
  }
  n183 = local write "Act. Step:"(w7) -> ()
  n184 = for {
    tunnel: "AxisControlSubPanelRefArray" -> [w355] mode=indexing
    tunnel: [w336] -> w8 mode=indexing
    tunnel: [w335] -> w6 mode=indexing
    tunnel: [w334] -> w5 mode=indexing
    tunnel: [w352] -> w3 mode=indexing
    i -> [w335]
    w334 = u16 0 ("AxisBaseAddr")
    w353 = T6 {"AxisName"="", "UnitsControl"=0, "AxisSlaveID"=0, "AxisBaseAddr"=0, "AxisMinSpeed"=0.0, "AxisMaxSpeed"=0.0}  # AxisConfiguration
    # "INIT axies data"
    n185 = invoke class="VI" method="Ctrl Val.Get"(reference=w355, "Control Name"="AxisName") -> (reference out=w345:refnum<vi>, error out=w343:errorcluster, "Get Control Value Variant"=w351:variant)  [unwired: 2 in, 1 out]
    n186 = invoke class="VI" method="Ctrl Val.Get"(reference=w345, error in=w343, "Control Name"="UnitsControl") -> (reference out=w344:refnum<vi>, error out=w342:errorcluster, "Get Control Value Variant"=w349:variant)  [unwired: 1 in, 1 out]
    n187 = invoke class="VI" method="Ctrl Val.Get"(reference=w344, error in=w342, "Control Name"="Max Velocity") -> ("Get Control Value Variant"=w347:variant)  [unwired: 1 in, 3 out]
    n188 = Variant To Data(type="0" ("Control Name"), Variant=w351) -> (data=w336:string)  [unwired: 1 in, 1 out]
    n189 = Variant To Data(type=u16 0, Variant=w349) -> (data=w339:u16)  [unwired: 1 in, 1 out]
    n190 = Variant To Data(type=u16 0, Variant=w347) -> (data=w338:u16)  [unwired: 1 in, 1 out]
    n191 = Bundle By Name(cluster=w353, "AxisName"=w336, "UnitsControl"=w339, "AxisSlaveID"=w335, "AxisBaseAddr"=w334, "AxisMinSpeed"=0.0, "AxisMaxSpeed"=w338) -> (w352:T6)
  }
  "AxisNames" <- w8
  "SlavesID" <- w6
  "AxisBaseAddr" <- w5
  n192 = while {
    stop <- FALSE stop-if-true
    # "CLose Panel event"
    n193 = event shown="[1] Panel Close" {
      selector: _ -> [_ _]
      dyn-events: _ -> [_ _]
      timeout: 20 -> [_ _]
      event Timeout {
        n194 = event-data() -> ()  [unwired: 1 in, 3 out]
      }
      event Panel Close {
        n195 = event-data() -> ()  [unwired: 1 in, 1 out]
        n196 = local read "Recipe example"() -> (w358:refnum<vi>)
        n197 = Stop(stop? (T)=TRUE) -> ()
        n198 = invoke class="VI" method="FP.Close"(reference=w358) -> (reference out=w359:refnum<vi>)  [unwired: 2 in, 2 out]
        n199 = invoke class="VI" method="Abort VI"(reference=w359) -> ()  [unwired: 2 in, 3 out]
      }
    }
  }
  n200 = control-ref of="SubPanel 1"() -> (w10:refnum<vi>)
  n201 = flat-sequence {
    tunnel: w10 -> [w376]
    tunnel: T1[] [{"Macro Type"=0, "Macro Name"="", "Macro Description"="", "M1_action_axis 1"=0, "M1_action_axis 2"=0, "M1_action_axis 3"=0, "M1_action_axis 4"=0, "M1_action_axis 5"=0, "M1_action_axis 6"=0, "M2_Axis"=0, "M2_Target_Pos"=0.0, "M2_Target_Vel"=0.0, "MoveModeControl"=1, "M3_1_Time"=0, "M3_Type"=0, "M3_2_wait_for_axis 1"=FALSE, "M3_2_wait_for_axis 2"=FALSE, "M3_2_wait_for_axis 3"=FALSE, "M3_2_wait_for_axis 4"=FALSE, "M3_2_wait_for_axis 5"=FALSE, "M3_2_wait_for_axis 6"=FALSE, "M3_3_mesage"="", "M3_3_wait_for_calib"=FALSE, "SelectedTargetCtrl"=1, "M5_select_action"=0}] ("Macro Table") -> [w371]
    tunnel: [w361] -> w4
    tunnel: w3 -> [w367]
    frame #0 {
      # "Load sub panel with recipe"
      n202 = Open VI Reference(vi path=path "Recipe example.vi") -> (vi reference=w373:refnum<vi>, error out=w372:errorcluster)  [unwired: 5 in]
      n203 = invoke class="VI" method="Ctrl Val.Set"(reference=w373, error in=w372, "Control Name"="Macro Table", "Value"=w371) -> (reference out=w370:refnum<vi>, error out=w369:errorcluster)  [unwired: 1 in, 3 out]
      n204 = invoke class="VI" method="Ctrl Val.Set"(reference=w370, error in=w369, "Control Name"="AxisConfigurations", "Value"=w367) -> (reference out=w366:refnum<vi>, error out=w363:errorcluster)  [unwired: 1 in, 3 out]
      n205 = local read "AllowCalib"() -> (w364:bool)
      n206 = invoke class="VI" method="Ctrl Val.Set"(reference=w366, error in=w363, "Control Name"="AllowCalib", "Value"=w364) -> (reference out=w361:refnum<vi>, error out=w362:errorcluster)  [unwired: 1 in, 3 out]
      n207 = invoke class="VI" method="Run VI"(reference=w361, error in=w362, "Wait until done"=FALSE ("Wait Until Done"), "Auto Dispose Ref"=FALSE ("Auto Dispose Reference")) -> (reference out=w377:refnum<vi>)  [unwired: 1 in, 4 out]
      n208 = invoke class="SubPnl" method="Insert VI"(reference=w376, "VI Ref"=w377) -> ()  [unwired: 2 in, 4 out]
    }
  }
  "Recipe example" <- w4
